vi "Initialize.vi"(8 "error in":errorcluster, 10 "parameters":variant, 11 "group in":refnum<class "device.lvclass">) -> (0 "error out":errorcluster, 2 "summary":T2[](array[typedef]), 3 "data value reference":T1)   [LabVIEW 2013, in "device.lvclass"]
doc: "This Vi initializes the data of a node its default state.\nThe object is not created inside of this ViI, beacuase it is created from a File depending on user selection."
uses:
  device.lvclass
  <vilib>/NI/Configuration Framework/Node/Summary.ctl
  <vilib>/NI/Configuration Framework/Node/NodeRef.ctl
  <vilib>/NI/Configuration Framework/Node/NISE_CEF_Node.lvclass
  device registry command.ctl
  device.lvclass/device.ctl
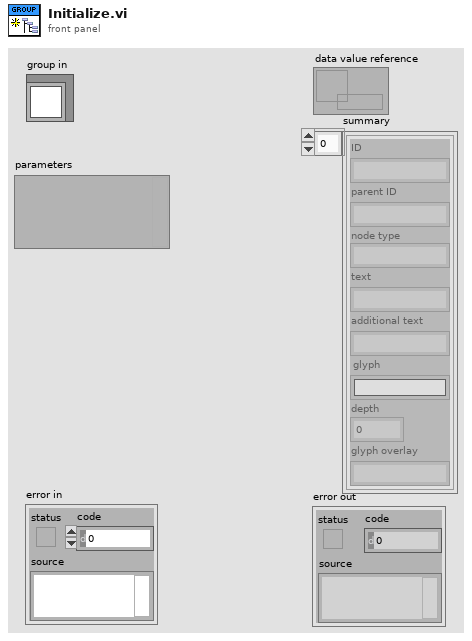
[diagram p1: front panel]
types:
  T1 = typedef "NISE_CEF_Node.lvclass/NodeRef.ctl" = refnum<data-value>
  T2 = typedef "NISE_CEF_Node.lvclass/Summary.ctl" = cluster{"ID":string, "parent ID":string, "node type":string, "text":string, "additional text":string, "glyph":string, "depth":i32, "glyph overlay":string}
  T3 = typedef "device.lvclass/device registry command.ctl" = enum16{"add device", "remove device", "get next available"}
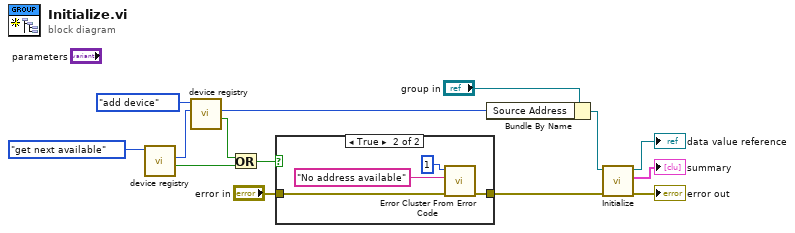
[diagram p0: block diagram]
diagram:
  n1 = call "device registry.vi"("command"=device_registry_command."get next available") -> ("Error?"=w4:bool, "device out"=w7:u8)  [unwired: 9 in]
  n2 = call "device registry.vi"("device"=w7, "command"=device_registry_command."add device") -> ("Error?"=w5:bool, "device out"=w6:u8)  [unwired: 8 in]
  n3 = Or(x=w5, y=w4) -> (x .or. y?=w3:bool)
  n4 = case shown="True" w3 {
    tunnel: "error in" -> [w15 w19]
    tunnel: [w15 w18] -> w1
    frame False {
    }
    frame True {
      n5 = call <vilib>:"Error Cluster From Error Code.vi"("error in (no error)"=w19, "error message (\"\")"="No address available" ("error message (\"\")"), "error code (0)"=1) -> ("error out"=w18:errorcluster)  [unwired: 6 in]
    }
  }
  n6 = Bundle By Name(cluster="group in", "Source Address"=w6) -> (w10:refnum<class "device.lvclass">)
  n7 = call-parent "Initialize.vi"("error in"=w1, "node in"=w10) -> ("error out"=→"error out":errorcluster, "summary"=→"summary":T2[], "data value reference"=→"data value reference":T1)  [unwired: 7 in]
